vi "IP_判断IP地址格式.vi"(8 "error in (no error)":errorcluster caption="错误输入（无错误）", 11 "IP地址":string) -> (0 "error out":errorcluster caption="错误输出", 2 "合法IP？":bool, 3 "IP地址 副本":string)   [LabVIEW 2018]
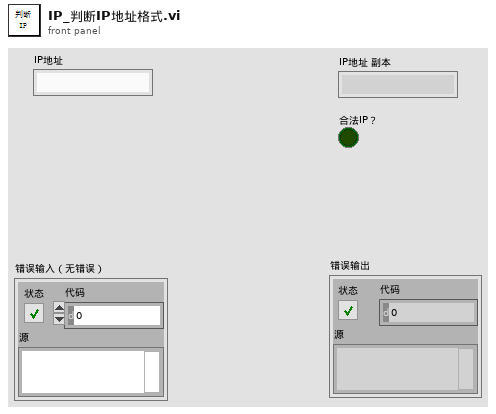
[diagram p1: front panel]
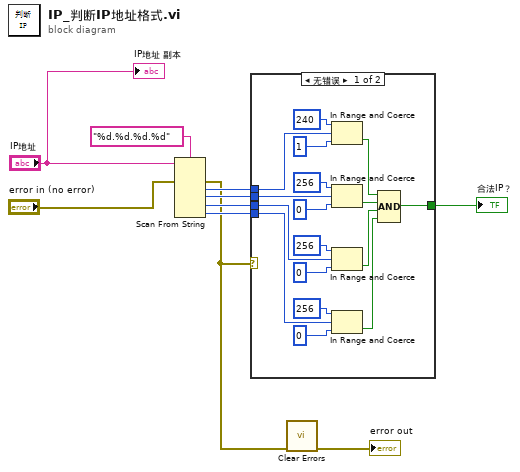
[diagram p0: block diagram]
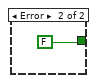
[diagram p2: hidden frame]
diagram:
  n1 = Scan From String(format string="%d.%d.%d.%d" ("格式字符串"), input string="IP地址", error in="error in (no error)") -> (error out=w2:errorcluster, output 1=w9:i32, output 2=w7:i32, output 3=w6:i32, output 4=w5:i32)  [unwired: 5 in, 2 out]
  n2 = case shown="无错误" w2 {
    tunnel: w9 -> [w27 _]
    tunnel: [w14 FALSE] -> w8
    tunnel: w7 -> [w13 _]
    tunnel: w6 -> [w12 _]
    tunnel: w5 -> [w11 _]
    frame No Error {
      n3 = In Range and Coerce(upper limit=240 ("上限"), x=w27, lower limit=1 ("下限")) -> (In Range?=w18:bool)  [unwired: 1 out]
      n4 = In Range and Coerce(upper limit=256 ("上限"), x=w13, lower limit=0 ("下限")) -> (In Range?=w17:bool)  [unwired: 1 out]
      n5 = In Range and Coerce(upper limit=256 ("上限"), x=w12, lower limit=0 ("下限")) -> (In Range?=w16:bool)  [unwired: 1 out]
      n6 = In Range and Coerce(upper limit=256 ("上限"), x=w11, lower limit=0 ("下限")) -> (In Range?=w15:bool)  [unwired: 1 out]
      n7 = Compound Arithmetic op=AND ("复合运算")(w18, w17, w16, w15) -> (w14:bool)
    }
    frame Error {
    }
  }
  "合法IP？" <- w8
  n8 = call <vilib>:"Clear Errors.vi"("error in (no error)"=w2) -> ("error out"=→"error out":errorcluster)  [unwired: 5 in, 1 out]
  "IP地址 副本" <- "IP地址"
